vi "Exercise6.vi"() -> ()   [LabVIEW 2019]
panel:
  out "millisecond timer value":u32
  out "?":bool
  out "5":bool
  out "4":bool
  out "3":bool
  out "2":bool
  out "miliseconds":u32
  out "1":bool
  # "FLAT"
  # "STACKED"
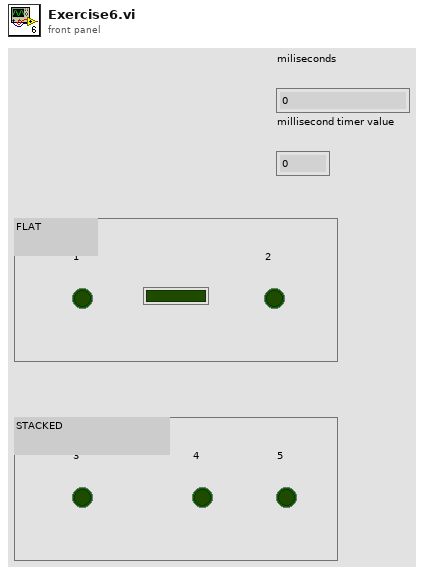
[diagram p1: front panel]
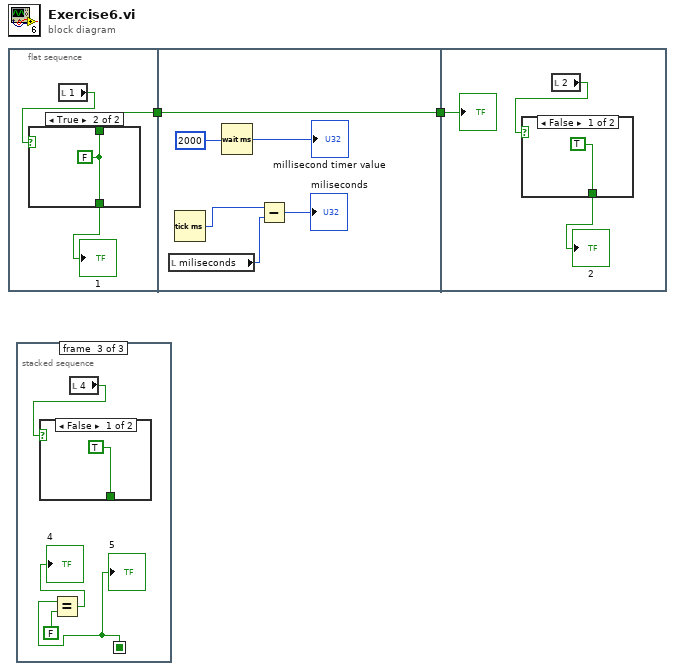
[diagram p0: block diagram]
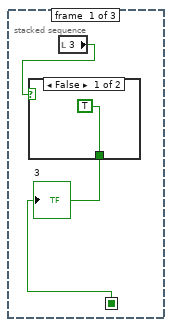
[diagram p2: hidden frame]
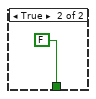
[diagram p3: hidden frame]
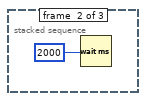
[diagram p4: hidden frame]
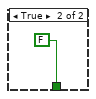
[diagram p5: hidden frame]
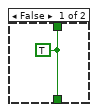
[diagram p6: hidden frame]
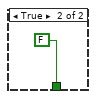
[diagram p7: hidden frame]
diagram:
  n1 = flat-sequence {
    tunnel: [w3] -> w1
    tunnel: [w12] -> w2
    tunnel: w1 -> [w12]
    tunnel: w2 -> [w14]
    frame #0 {
      n2 = local read "1"() -> (w5:bool)
      n3 = case shown="True" w5 {
        tunnel: [w6 w7] -> w4
        tunnel: [w6 w7] -> w3
        frame False {
          w6 = TRUE
        }
        frame True {
          w7 = FALSE
        }
      }
      "1" <- w4
    }
    frame #1 {
      n4 = local read "miliseconds"() -> (w10:u32)
      n5 = Tick Count (ms)() -> (millisecond timer value=w9:u32)
      n6 = Wait (ms)(milliseconds to wait=u32 2000 ("millisecond timer value")) -> (millisecond timer value=→"millisecond timer value":u32)
      n7 = Subtract(x=w9, y=w10) -> (x-y=→"miliseconds":u32)
    }
    frame #2 {
      n8 = local read "2"() -> (w16:bool)
      n9 = case shown="False" w16 {
        tunnel: [TRUE FALSE] -> w15
        frame False {
        }
        frame True {
        }
      }
      "2" <- w15
      "?" <- w14
    }
  }
  n10 = stacked-sequence {
    seq-local: [w19 _ _] -> [_ _ w24]
    frame #0 {
      n11 = local read "3"() -> (w20:bool)
      n12 = case shown="False" w20 {
        tunnel: [TRUE FALSE] -> w19
        frame False {
        }
        frame True {
        }
      }
      "3" <- w19
    }
    frame #1 {
      n13 = Wait (ms)(milliseconds to wait=u32 2000 ("millisecond timer value")) -> ()  [unwired: 1 out]
    }
    frame #2 {
      n14 = Equal?(x=w24, y=FALSE) -> (x = y?=→"4":bool)
      n15 = local read "4"() -> (w27:bool)
      n16 = case shown="False" w27 {
        tunnel: [TRUE FALSE] -> _
        frame False {
        }
        frame True {
        }
      }
      "5" <- w24
    }
  }
